vi "MikolajczykMarcin_kolokwium1.vi"() -> ()   [LabVIEW 2025]
panel:
  out "x+y":dbl
  out "t0 2":dbl
  in  "Temperatura":enum16{"70", "80", "90", "100"}(ring)
  in  "t0":dbl
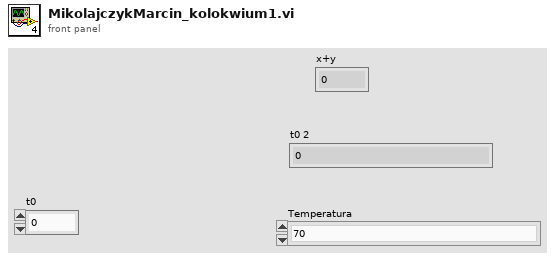
[diagram p1: front panel]
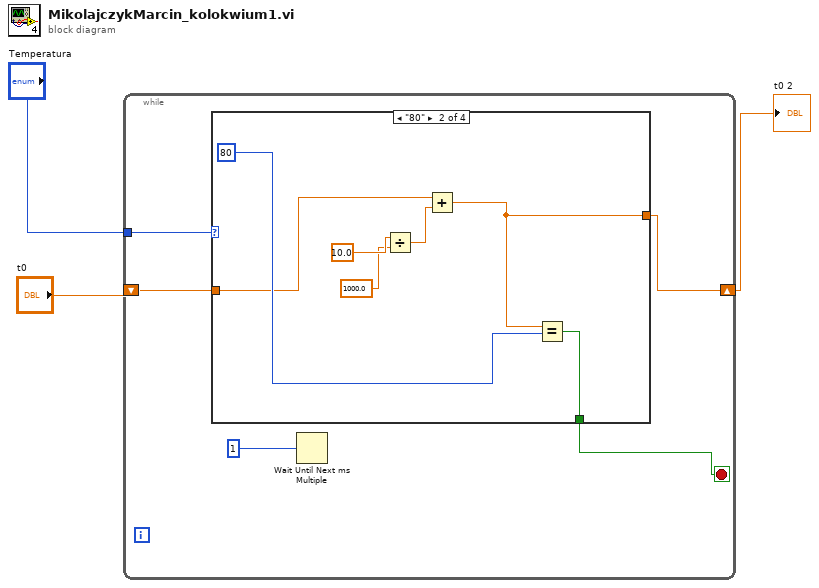
[diagram p0: block diagram]
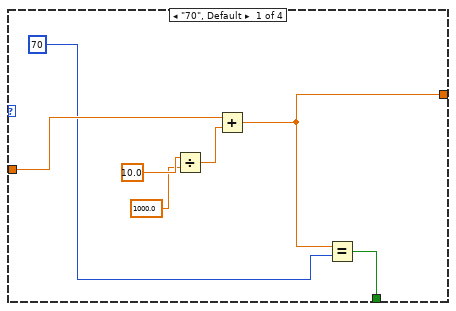
[diagram p2: hidden frame]
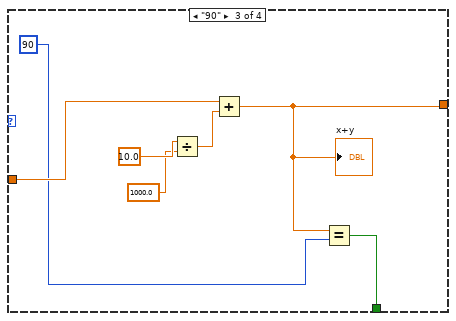
[diagram p3: hidden frame]
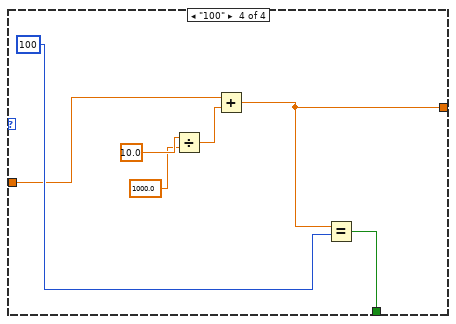
[diagram p4: hidden frame]
diagram:
  n1 = while {
    tunnel: "Temperatura" -> [w8]
    shift-right: [w6] -> w1
    shift-left: "t0" -> [w5]
    stop <- w7 stop-if-true
    n2 = case shown="\"80\"" w8 {
      tunnel: [w10 w18 w24 w32] -> w7
      tunnel: [w9 w17 w23 w31] -> w6
      tunnel: w5 -> [w12 w16 w26 w30]
      frame "70", Default {
        n3 = Divide(x=10.0 ("y"), y=1000.0) -> (x/y=w13:dbl)
        n4 = Add(x=w12, y=w13) -> (x+y=w9:dbl)
        n5 = Equal?(x=w9, y=70) -> (x = y?=w10:bool)
      }
      frame "80" {
        n6 = Divide(x=10.0 ("y"), y=1000.0) -> (x/y=w20:dbl)
        n7 = Add(x=w16, y=w20) -> (x+y=w17:dbl)
        n8 = Equal?(x=w17, y=80) -> (x = y?=w18:bool)
      }
      frame "90" {
        n9 = Divide(x=10.0 ("y"), y=1000.0) -> (x/y=w27:dbl)
        n10 = Add(x=w26, y=w27) -> (x+y=w23:dbl)
        "x+y" <- w23
        n11 = Equal?(x=w23, y=90) -> (x = y?=w24:bool)
      }
      frame "100" {
        n12 = Divide(x=10.0 ("y"), y=1000.0) -> (x/y=w34:dbl)
        n13 = Add(x=w30, y=w34) -> (x+y=w31:dbl)
        n14 = Equal?(x=w31, y=100) -> (x = y?=w32:bool)
      }
    }
    n15 = Wait Until Next ms Multiple(millisecond multiple=u32 1) -> ()  [unwired: 1 out]
  }
  "t0 2" <- w1
